vi "Write Sections.vi"(8 "error in (no error)":errorcluster, 10 "Sections":refnum<class "Section.lvclass">[](array[class]), 11 "Configuration in":refnum<class "Configuration.lvclass">) -> (0 "error out":errorcluster, 3 "Configuration out":refnum<class "Configuration.lvclass">)   [LabVIEW 2015, in "Configuration.lvlib" / "Configuration.lvclass"]
doc: "Write sections to class private data."
uses:
  Configuration.lvclass
  Section/Section.lvclass
  Configuration.lvclass/Configuration.ctl
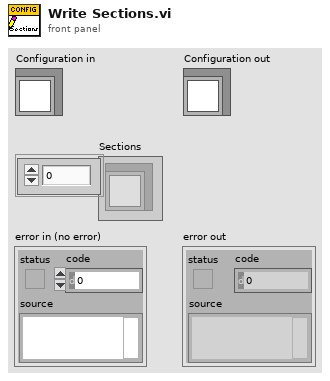
[diagram p1: front panel]
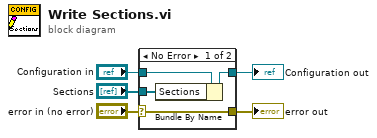
[diagram p0: block diagram]
diagram:
  n1 = case shown="No Error" "error in (no error)" {
    selector: "error in (no error)" -> [w9 w10]
    tunnel: [w9 w10] -> w4
    tunnel: [w7 w11] -> w2
    tunnel: "Configuration in" -> [w8 w11]
    tunnel: "Sections" -> [w6 _]
    frame No Error {
      n2 = Bundle By Name(cluster=w8, "Sections"=w6) -> (w7:refnum<class "Configuration.lvclass">)
    }
    frame Error {
    }
  }
  "error out" <- w4
  "Configuration out" <- w2
